vi "Get Comparison Test Settings.vi"(8 "error in (no error)":errorcluster, 11 "Data Channel Ref In":T1=18446744073709551615 format="%.0x") -> (0 "error out":errorcluster, 2 "Data Channel Settings":T2, 3 "Data Channel Ref Out":T1=18446744073709551615 format="%.0x")   [LabVIEW 2019, in "Instrument Addon Scripting API Channels Unit Tests.lvclass"]
uses:
  Instrument Addon Scripting API Channels Unit Tests.lvclass
  APIs/Scripting API/TypeDefs/Array Comparison Settings.ctl
  APIs/Scripting API/TypeDefs/Array Element.ctl
  <vilib>/NI VeriStand/Custom Device API/Custom Device Item Ref.ctl
  <vilib>/NI VeriStand/Custom Device API/Get Item Property (String).vi
  <vilib>/NI VeriStand/Custom Device API/Custom Device API.lvlib
  APIs/Scripting API/Instrument Addon Scripting API.lvlib
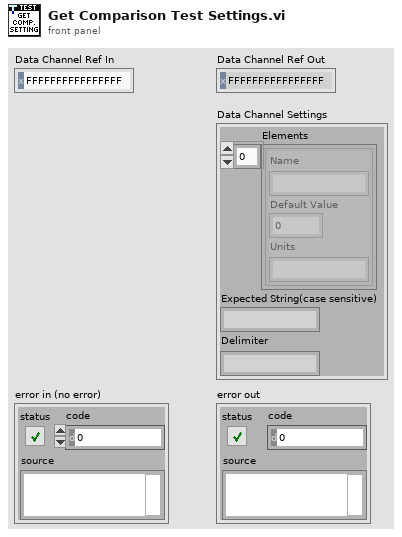
[diagram p1: front panel]
types:
  T1 = typedef "Custom Device API.lvlib/Custom Device Item Ref.ctl" = u64
  T2 = typedef "Instrument Addon Scripting API.lvlib/Array Comparison Settings.ctl" = cluster{"Elements":T3[], "Expected String(case sensitive)":string, "Delimiter":string}
  T3 = typedef "Instrument Addon Scripting API.lvlib/Array Element.ctl" = cluster{"Name":string, "Default Value":dbl, "Units":string}
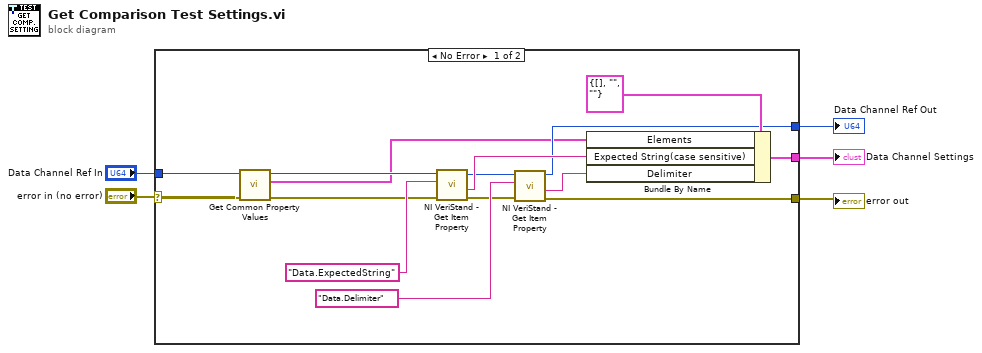
[diagram p0: block diagram]
diagram:
  n1 = case shown="No Error" "error in (no error)" {
    selector: "error in (no error)" -> [w11 w22]
    tunnel: "Data Channel Ref In" -> [w10 w21]
    tunnel: [w20 _] -> w5
    tunnel: [w17 w22] -> w4
    tunnel: [w7 w21] -> w2
    frame No Error {
      n2 = call "Get Common Property Values.vi"("Error In"=w11, "Data Channel  Ref in"=w10) -> ("error out"=w8:errorcluster, "Array Out"=w6:T3[], "Data Channel Ref Out"=w9:u64)  [unwired: 7 in]
      n3 = call-poly <vilib>:"NI VeriStand - Get Item Property.vi"("error in (no error)"=w8, "Property Name"="Data.ExpectedString", "Item Ref in"=w9) -> ("error out"=w13:errorcluster, "Value"=w19:string, "Item Ref out"=w14:T1)  [unwired: 5 in, 1 out]
      n4 = call-poly <vilib>:"NI VeriStand - Get Item Property.vi"("error in (no error)"=w13, "Property Name"="Data.Delimiter", "Item Ref in"=w14) -> ("error out"=w17:errorcluster, "Value"=w16:string, "Item Ref out"=w7:T1)  [unwired: 5 in, 1 out]
      n5 = Bundle By Name(cluster=T2 {"Elements"=[], "Expected String(case sensitive)"="", "Delimiter"=""} ("Settings"), "Elements"=w6, "Expected String(case sensitive)"=w19, "Delimiter"=w16) -> (w20:T2)
    }
    frame Error {
    }
  }
  "Data Channel Settings" <- w5
  "error out" <- w4
  "Data Channel Ref Out" <- w2
